vi "Get IO Level.vi"(10 "iLevel":i32, 11 "index":i32) -> (2 "iLevel out":i32, 3 "function return":u32)   [LabVIEW 2018, in "AndorSDK.lvlib"]
doc: "EXPNETTYPE unsigned int WINAPI GetIOLevel(int index, int * iLevel);"
uses:
  AndorSDK.lvlib
  ATMCD32D.dll
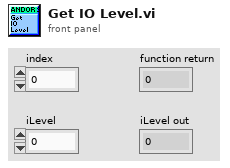
[diagram p1: front panel]
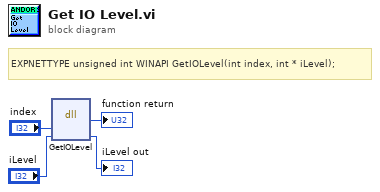
[diagram p0: block diagram]
diagram:
  # "EXPNETTYPE unsigned int WINAPI GetIOLevel(int index, int * iLevel);"
  n1 = dll-call lib="PTH2babs E\nPersönliches02 - Arbeit03-HiwijobsLabviewCodelibANDOR\tAndor SDK\nATMCD32D.*" fn="GetIOLevel"("index"="index", "iLevel"="iLevel") -> (→"function return":u32, "iLevel"=→"iLevel out":i32)  [unwired: 4 in, 2 out]
